vi "FFTLowFreqFilter.vi"(11 "Power Spectrum / PSD":cluster{"f0":dbl, "df":dbl, "magnitude":dbl[]}) -> (1 "df":dbl, 2 "f0":dbl, 3 "Power FFT":cluster{"f0":dbl, "df":dbl, "magnitude":dbl[]}(graph), 4 "Max Freq (Hz)":dbl, 5 "Raw magnitude":dbl[](array[numeric]), 6 "Filtered output array":dbl[](array[numeric]))   [LabVIEW 2015]
panel:
  out "max index(es)":i32
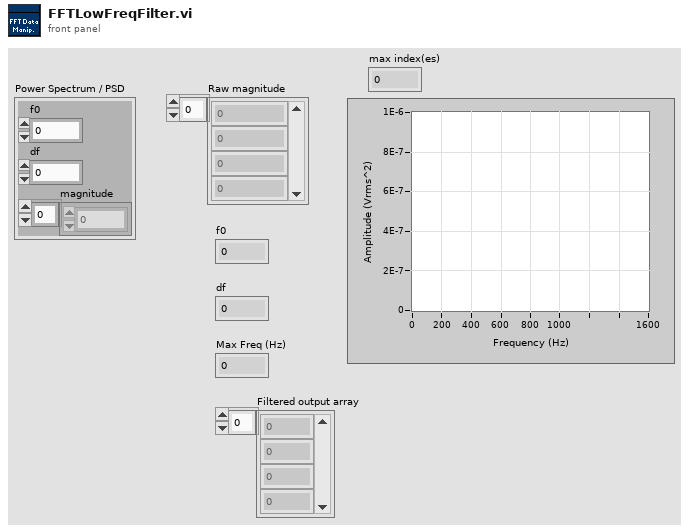
[diagram p1: front panel]
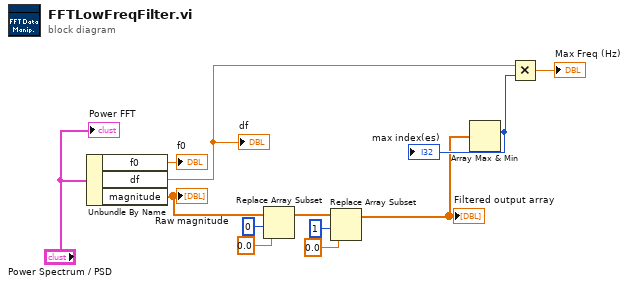
[diagram p0: block diagram]
diagram:
  n1 = Unbundle By Name("Power Spectrum / PSD") -> ("f0"=→"f0":dbl, "df"=w11:dbl, "magnitude"=w8:dbl[])
  "df" <- w11
  "Raw magnitude" <- w8
  n2 = Replace Array Subset(array=w8, new element=0.0 ("new element/subarray"), index=0) -> (w9:dbl[])
  n3 = Replace Array Subset(array=w9, new element=0.0 ("new element/subarray"), index=1) -> (w1:dbl[])
  "Filtered output array" <- w1
  n4 = Array Max & Min(array=w1) -> (max index (indices)=w10:i32)  [unwired: 3 out]
  "max index(es)" <- w10
  n5 = Multiply(x=w11, y=w10) -> (x*y=→"Max Freq (Hz)":dbl)
  "Power FFT" <- "Power Spectrum / PSD"
